vi "Panel from Subpanel.vi"(8 "error in (no error)":errorcluster, 10 "Sub Panel":refnum<vi>, 11 "PanelManager in":refnum<class "PanelManager.lvclass">) -> (0 "error out":errorcluster, 1 "Has Panel?":bool, 2 "Panel":refnum<class "Panel.lvclass">, 3 "PanelManager out":refnum<class "PanelManager.lvclass">)   [LabVIEW 2018, in "OOPanel.lvlib" / "PanelManager.lvclass"]
uses:
  PanelManager.lvclass
  Panel/Panel.lvclass
  PanelManager.lvclass/PanelManager.ctl
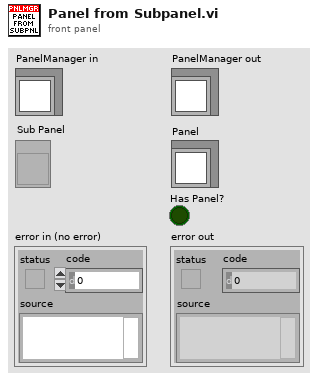
[diagram p1: front panel]
types:
  T1 = typedef "OOPanel.lvlib/PanelManager.lvclass/Ref Data.ctl" = cluster{"Panels":T2, "Subpanel Map":T3}
  T2 = typedef "OOPanel.lvlib/PanelManager.lvclass/Panels.ctl" = cluster{"Names":string[], "Instances":refnum<class "Panel.lvclass">[]}
  T3 = typedef "OOPanel.lvlib/PanelManager.lvclass/SubPanel Map.ctl" = cluster{"SubPanels":refnum<vi>[], "Panels":refnum<class "Panel.lvclass">[]}
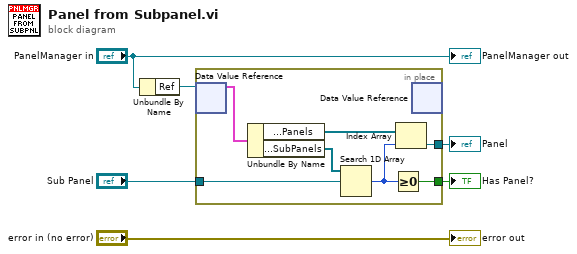
[diagram p0: block diagram]
diagram:
  n1 = Unbundle By Name("PanelManager in") -> ("Ref"=w5:refnum<data-value>)
  n2 = in-place {
    in-place-border: "Sub Panel" -> [w12]
    in-place-border: [w8] -> w2
    in-place-border: [w7] -> w1
    n3 = in-place-dvr #1(w5) -> (w13:T1)  [unwired: 1 out]
    n4 = Unbundle By Name(w13) -> ("Subpanel Map.Panels"=w10:refnum<class "Panel.lvclass">[], "Subpanel Map.SubPanels"=w11:refnum<vi>[])
    n5 = Search 1D Array(1D array=w11, element=w12) -> (index of element=w9:i32)  [unwired: 1 in]
    n6 = Greater Or Equal To 0?(x=w9) -> (x >= 0?=w7:bool)
    n7 = Index Array(array=w10, index=w9) -> (element=w8:refnum<class "Panel.lvclass">)
    n8 = in-place-dvr #1() -> ()  [unwired: 1 in, 2 out]
  }
  "Panel" <- w2
  "Has Panel?" <- w1
  "error out" <- "error in (no error)"
  "PanelManager out" <- "PanelManager in"
